vi "Example_DIO_DWG_file.vi"() -> ()   [LabVIEW 2013]
uses:
  <vilib>/Signadyne/Wave/base/waveformLoadWave.vi
  Instance          10 28Saved   Example_DIO_DWG_file .vi
panel:
  in  "Waveform file":string
  in  "End Line":i32=19
  in  "Start Line":i32=16
  in  "Slot":i32=4
  out "ConfigBus Status":errorcluster
  out "DirConfig":errorcluster
  out "Bus value":i64
  out "Close Status":errorcluster
  in  "Stop Loop":bool
  out "Open Status":errorcluster
  in  "Part Number":string="SD-PXE-DIO-H0002-1G"
  # "Output&Input Bus"
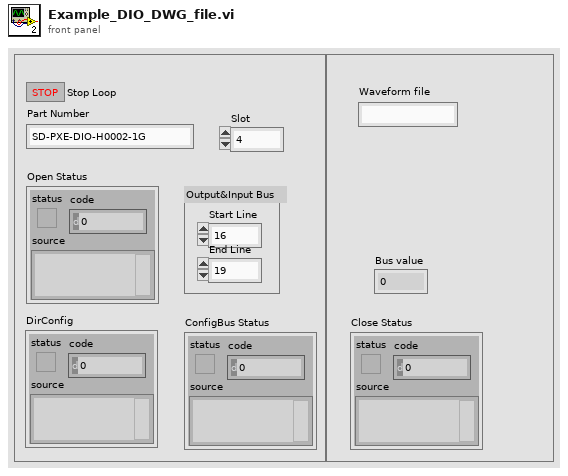
[diagram p1: front panel]
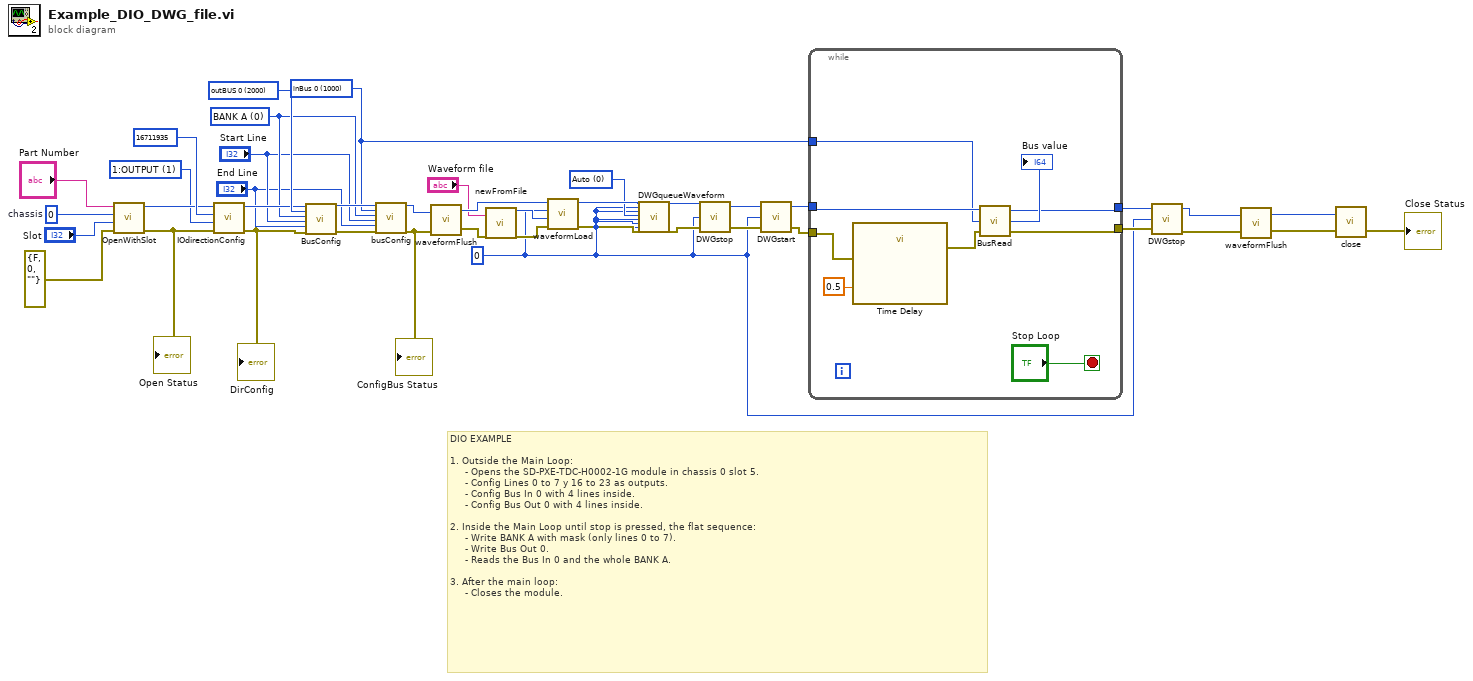
[diagram p0: block diagram]
diagram:
  w1 = 1000 items=["inBus 0"=1000, "inBus 1"=1001, "outBus 0"=2000, "outBus 1"=2001] ("nBus")
  w22 = 0 items=["Auto", "VI/HVI", "External"] ("triggerMode")
  w13 = 0 ("waveformNumber")
  w4 = 0 items=["BANK A"=0, "BANK B"=1, "BANK B:A"=3000] ("nPort")
  w34 = 2000 items=["inBus 0"=1000, "outBUS 0"=2000] ("nBus")
  w35 = u16 1 items=["0:INPUT", "1:OUTPUT"] ("direction")
  w39 = 0  # chassis
  # "DIO EXAMPLE\n\n1. Outside the Main Loop:\n     - Opens the SD-PXE-TDC-H0002-1G module in chassis 0 slot 5.\n     - Config Lines 0 to 7 y 16 to 23 as outputs.\n     - Config Bus In 0 with 4 lines inside.\n     - Config Bus Out 0 with 4 lines inside.\n\n2. Inside the Main Loop until stop is pressed, the flat sequence:\n     - Write BANK A with mask (only lines 0 to 7).\n     - Write Bus Out 0.\n     - Reads the Bus In 0 and the whole BANK A.\n\n3. After the main loop:\n     - Closes the module."
  n1 = call <vilib>:"OpenWithSlot.vi"("errorIn"=errorcluster {"status"=FALSE, "code"=0, "source"=""}, "nSlot"="Slot", "nChassis"=w39, "partNumber"="Part Number") -> ("errorOut"=w38:errorcluster, "moduleID"=w36:i32)  [unwired: 2 in]
  "Open Status" <- w38
  n2 = call <vilib>:"IOdirectionConfig.vi"("errorIn"=w38, "direction"=w35, "lineMask"=i64 16711935, "moduleID"=w36) -> ("errorOut"=w31:errorcluster, "moduleIDOut"=w30:i32)  [unwired: 2 in]
  "DirConfig" <- w31
  n3 = call <vilib>:"BusConfig.vi"("moduleID"=w30, "nBus"=w34, "port"=w4, "start"="Start Line", "end"="End Line", "errorIn"=w31) -> ("moduleIDOut"=w5:i32, "errorOut"=w6:errorcluster)  [unwired: 12 in]
  n4 = call <vilib>:"busConfig.vi"("moduleID"=w5, "nBus"=w1, "port"=w4, "start"="Start Line", "end"="End Line", "errorIn"=w6) -> ("moduleIDOut"=w8:i32, "errorOut"=w7:errorcluster)  [unwired: 12 in]
  "ConfigBus Status" <- w7
  n5 = call <vilib>:"waveformFlush.vi"("errorIn"=w7, "moduleID"=w8) -> ("errorOut"=w26:errorcluster, "moduleIDOut"=w27:i32)
  n6 = call <vilib>:"newFromFile.vi"("waveformFile"="Waveform file", "errorIn"=w26) -> ("waveformID"=w28:i32, "errorOut"=w29:errorcluster)  [unwired: 16 in]
  n7 = call-poly <vilib>:"waveformLoad.vi"("errorIn"=w29, "waveformID"=w28, "waveformNumber"=w13, "moduleID"=w27) -> ("errorOut"=w23:errorcluster, "moduleIDOut"=w24:i32)  [unwired: 5 in, 1 out]
  n8 = call <vilib>:"DWGqueueWaveform.vi"("moduleID"=w24, "DWG"=w13, "waveformNumber"=w13, "triggerMode"=w22, "startDelay"=w13, "cycles"=w13, "prescaler"=w13, "errorIn"=w23) -> ("moduleIDOut"=w20:i32, "errorOut"=w21:errorcluster)  [unwired: 18 in]
  n9 = call <vilib>:"DWGstop.vi"("errorIn"=w21, "DWG"=w13, "moduleID"=w20) -> ("errorOut"=w19:errorcluster, "moduleIDOut"=w18:i32)  [unwired: 1 in]
  n10 = call <vilib>:"DWGstart.vi"("errorIn"=w19, "DWG"=w13, "moduleID"=w18) -> ("errorOut"=w17:errorcluster, "moduleIDOut"=w16:i32)  [unwired: 1 in]
  n11 = while {
    tunnel: [w43] -> w14
    tunnel: [w44] -> w15
    tunnel: w16 -> [w45]
    tunnel: w17 -> [w46]
    tunnel: w1 -> [w42]
    stop <- "Stop Loop" stop-if-true
    n12 = call "Time Delay"("error in (no error)"=w46, "Delay Time (s)"=0.5) -> ("error out"=w48:errorcluster)  [unwired: 9 in]
    n13 = call <vilib>:"BusRead.vi"("errorIn"=w48, "inBus"=w42, "moduleID"=w45) -> ("errorOut"=w44:errorcluster, "portValue"=→"Bus value":i64, "moduleIDOut"=w43:i32)
  }
  n14 = call <vilib>:"DWGstop.vi"("errorIn"=w15, "DWG"=w13, "moduleID"=w14) -> ("errorOut"=w9:errorcluster, "moduleIDOut"=w10:i32)  [unwired: 1 in]
  n15 = call <vilib>:"waveformFlush.vi"("errorIn"=w9, "moduleID"=w10) -> ("errorOut"=w12:errorcluster, "moduleIDOut"=w11:i32)
  n16 = call <vilib>:"close.vi"("errorIn"=w12, "moduleID"=w11) -> ("errorOut"=→"Close Status":errorcluster)  [unwired: 1 in]
